vi "Keithley DMM6500 DAQ6500 Series Measure 4W Resistance With Offset Compensation.vi"() -> ()   [LabVIEW 2020]
doc: "This example shows how to configure DMM to measure 4W resistance."
uses:
  <instrlib>/Keithley DMM6500 DAQ6500 Series/Public/Data/Read (Single Point).vi
  <instrlib>/Keithley DMM6500 DAQ6500 Series/Keithley DMM6500 DAQ6500 Series.lvlib
panel:
  in  "Offset Compensate Mode(2: Auto)":i32(ring)=2 items=["Disabled", "Enabled", "Auto"]
  in  "Auto Zero (0: Enable)":u32(ring) items=["Enable", "Disable", "Once"]
  in  "Power Line Cycle (10)":dbl=10.0
  out "Measurement":dbl
  in  "Channel List (\"101\")":string="101"
  in  "VISA resource name":refnum<visa-resource-name>
  # "(c) 2018-2022 National Instruments.  ALL RIGHTS RESERVED."
  # "This example VI demonstrates how to use the DMM6500 or DAQ6500 Series to accurately measure a resistance device via front or rear terminals. To obtain the best results, the 4-wire (Kelvin) measurement function and offset compensation are used for this test.\nIf it's for DMM the Channel List control will take no effect."
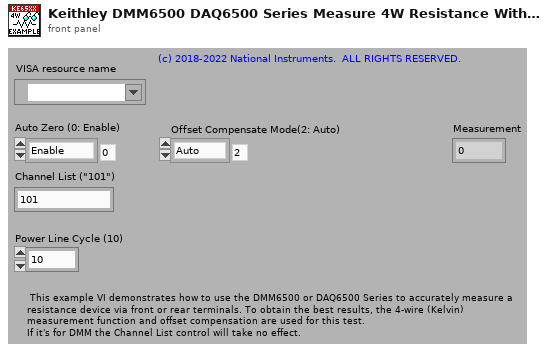
[diagram p1: front panel]
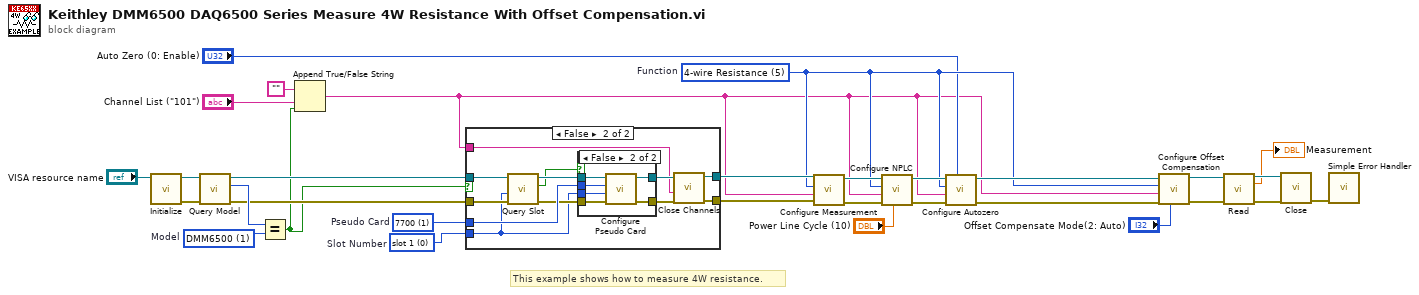
[diagram p0: block diagram]
diagram:
  w3 = 0 items=["slot 1", "slot 2"]  # Slot Number
  w2 = 1 items=["0", "7700", "7701", "7702", "7703", "7705", "7706", "7707", "7708", "7709", "7710", "7711", "7712"]  # Pseudo Card
  w9 = 5 items=[" Voltage DC", "Voltage AC", "Current DC", "Current AC", "Resistance", "4-wire Resistance", "Diode", "Capacitance", "Temperature", "Continuity", "Frequency", "Period", "Voltage Ratio", "Digitize Voltage", "Digitize Current"]  # Function
  w14 = 1 items=["", "DMM6500", "DAQ6510"]  # Model
  # "This example shows how to measure 4W resistance."
  n1 = call <instrlib>:"Initialize.vi"("VISA resource name"="VISA resource name") -> ("error out"=w11:errorcluster, "VISA resource name out"=w10:refnum<visa-resource-name>)  [unwired: 9 in]
  n2 = call <instrlib>:"Query Model.vi"("error in (no error)"=w11, "VISA resource name"=w10) -> ("error out"=w13:errorcluster, "Model"=w15:i32, "VISA resource name out"=w12:refnum<visa-resource-name>)  [unwired: 7 in]
  n3 = Equal?(x=w15, y=w14) -> (x = y?=w4:bool)
  n4 = Append True/False String(1:w4, 2:"Channel List (\"101\")", 3:"") -> (0:w6:string)  [unwired: 1 in]
  n5 = case shown="False" w4 {
    tunnel: w2 -> [_ w40]
    tunnel: w3 -> [_ w35]
    tunnel: w12 -> [w33 w45]
    tunnel: w13 -> [w32 w37]
    tunnel: [w33 w43] -> w19
    tunnel: [w32 w41] -> w18
    tunnel: w6 -> [_ w39]
    frame True {
    }
    frame False {
      n6 = call <instrlib>:"Query Slot.vi"("error in (no error)"=w37, "Slot Number(0: slot 1)"=w35, "VISA resource name"=w45) -> ("error out"=w36:errorcluster, "Real Card In Slot"=w34:bool, "VISA resource name out"=w38:refnum<visa-resource-name>)  [unwired: 6 in]
      n7 = case shown="False" w34 {
        tunnel: [w47 w53] -> w44
        tunnel: [w46 w52] -> w42
        tunnel: w40 -> [_ w51]
        tunnel: w38 -> [w47 w50]
        tunnel: w36 -> [w46 w49]
        tunnel: w35 -> [_ w48]
        frame True {
        }
        frame False {
          n8 = call <instrlib>:"Configure Pseudo Card.vi"("error in (no error)"=w49, "Slot Number (0: slot1)"=w48, "Pseudo Card (0:No pseudocard)"=w51, "VISA resource name"=w50) -> ("error out"=w52:errorcluster, "VISA resource name out"=w53:refnum<visa-resource-name>)  [unwired: 6 in]
        }
      }
      n9 = call <instrlib>:"Close Channels.vi"("error in (no error)"=w42, "Channel List(\"\")"=w39, "VISA resource name"=w44) -> ("error out"=w41:errorcluster, "VISA resource name out"=w43:refnum<visa-resource-name>)  [unwired: 7 in]
    }
  }
  n10 = call <instrlib>:"Configure Measurement.vi"("error in (no error)"=w18, "Channel List(\"\")"=w6, "Function (0: Voltage DC)"=w9, "VISA resource name"=w19) -> ("error out"=w16:errorcluster, "VISA resource name out"=w17:refnum<visa-resource-name>)  [unwired: 6 in]
  n11 = call <instrlib>:"Configure NPLC.vi"("Power Line Cycle (1)"="Power Line Cycle (10)", "error in (no error)"=w16, "Channel List(\"\")"=w6, "Function (0: Voltage DC)"=w9, "VISA resource name"=w17) -> ("error out"=w28:errorcluster, "VISA resource name out"=w29:refnum<visa-resource-name>)  [unwired: 5 in]
  n12 = call <instrlib>:"Configure Autozero.vi"("Auto Zero (0: Enable)"="Auto Zero (0: Enable)", "error in (no error)"=w28, "Channel List(\"\")"=w6, "Function (0: Voltage DC)"=w9, "VISA resource name"=w29) -> ("error out"=w22:errorcluster, "VISA resource name out"=w23:refnum<visa-resource-name>)  [unwired: 5 in]
  n13 = call <instrlib>:"Configure Offset Compensation.vi"("Offset Compensate Mode(2: Auto)"="Offset Compensate Mode(2: Auto)", "error in (no error)"=w22, "Channel List(\"\")"=w6, "Function (5: 4-wire resistance)"=w9, "VISA resource name"=w23) -> ("error out"=w20:errorcluster, "VISA resource name out"=w21:refnum<visa-resource-name>)  [unwired: 5 in]
  n14 = call-poly <instrlib>:"Read.vi"("VISA resource name"=w21, "error in (no error)"=w20) -> ("VISA resource name out"=w26:refnum<visa-resource-name>, "Measurement"=→"Measurement":dbl, "error out"=w27:errorcluster)  [unwired: 11 in]
  n15 = call <instrlib>:"Close.vi"("error in (no error)"=w27, "VISA resource name"=w26) -> ("error out"=w31:errorcluster)  [unwired: 9 in]
  n16 = call <vilib>:"Simple Error Handler.vi"("error in (no error)"=w31) -> ()  [unwired: 4 in, 5 out]
